vi "TCP Read.vi"(8 "error in (no error)":errorcluster, 10 "timeout ms (25000)":i32, 11 "TCP Network Connection in":refnum<k5>) -> (0 "error out":errorcluster, 2 "Message data out":string, 3 "TCP Network Connection out":refnum<k5>)   [LabVIEW 2014]
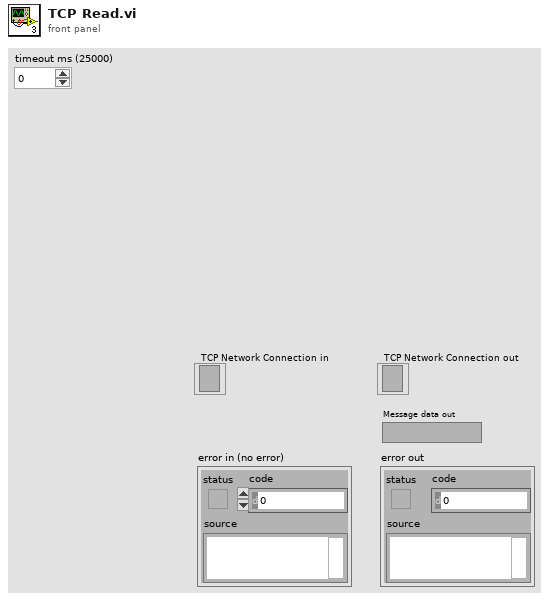
[diagram p1: front panel]
types:
  T1 = enum16{"Standard", "Buffered", "CRLF", "Immediate"}
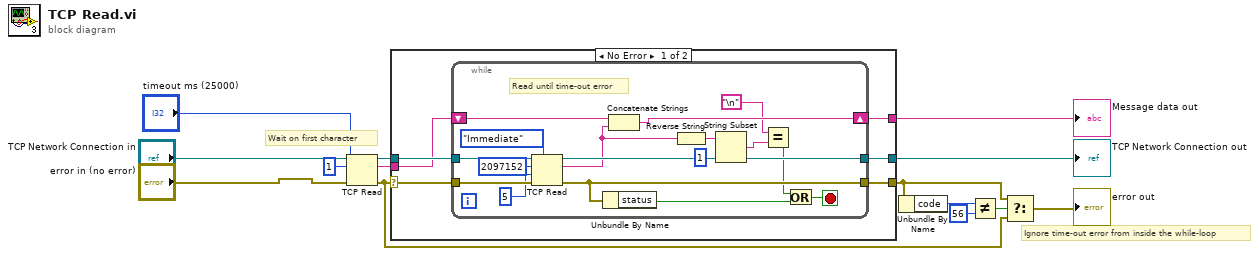
[diagram p0: block diagram]
diagram:
  # "Ignore time-out error from inside the while-loop"
  # "Wait on first character"
  n1 = TCP Read(connection ID="TCP Network Connection in", bytes to read=1, error in (no error)="error in (no error)", 9:"timeout ms (25000)") -> (connection ID out=w12:refnum<k5>, data out=w11:string, error out=w4:errorcluster)  [unwired: 1 in]
  n2 = case shown="No Error" w4 {
    selector: w4 -> [w15 w38]
    tunnel: [w20 w40] -> w14
    tunnel: [w19 w38] -> w5
    tunnel: w12 -> [w18 w40]
    tunnel: w11 -> [w17 w39]
    tunnel: [w16 w39] -> w10
    frame No Error {
      n3 = while {
        tunnel: [w37] -> w20
        tunnel: [w24] -> w19
        tunnel: w18 -> [w35]
        tunnel: w15 -> [w34]
        shift-right: [w31] -> w16
        shift-left: w17 -> [w32]
        stop <- w23 stop-if-true
        # "Read until time-out error"
        n4 = TCP Read(connection ID=w35, bytes to read=2097152, error in (no error)=w34, 7:T1."Immediate" ("mode (standard)"), 9:5 ("timeout ms (25000)")) -> (connection ID out=w37:refnum<k5>, data out=w28:string, error out=w24:errorcluster)
        n5 = Unbundle By Name(w24) -> ("status"=w21:bool)
        n6 = Concatenate Strings(w32, w28) -> (w31:string)
        n7 = Reverse String(1:w28) -> (0:w29:string)
        n8 = String Subset(string=w29, length (rest)=1 ("length (rest)")) -> (substring=w26:string)  [unwired: 1 in]
        n9 = Equal?(x="\n", y=w26) -> (x = y?=w22:bool)
        n10 = Or(x=w22, y=w21) -> (x .or. y?=w23:bool)
      }
    }
    frame Error {
    }
  }
  "Message data out" <- w10
  "TCP Network Connection out" <- w14
  n11 = Unbundle By Name(w5) -> ("code"=w9:i32)
  n12 = Not Equal?(x=w9, y=56) -> (x != y?=w7:bool)
  n13 = Select(t=w5, s=w7, f=w4) -> (s? t:f=→"error out":errorcluster)
